vi "Z_plant.vi"(4 "u":dbl format="%#_13g") -> (1 "y":dbl)   [LabVIEW 2015]
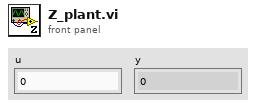
[diagram p1: front panel]
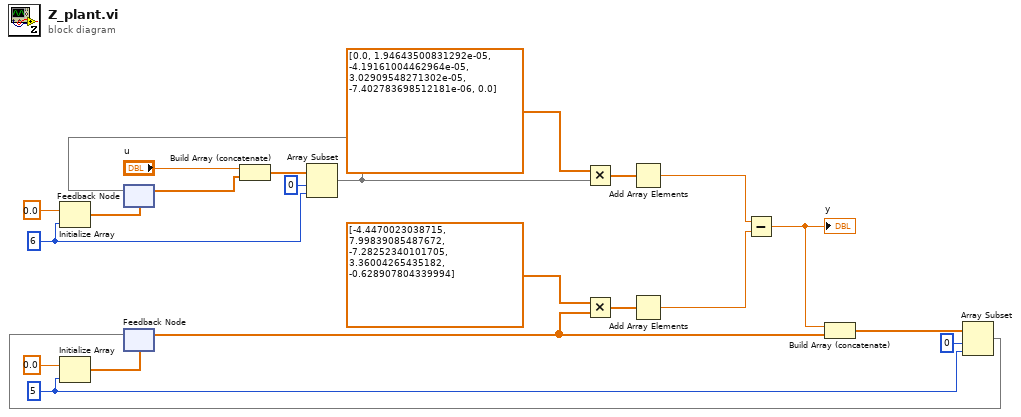
[diagram p0: block diagram]
diagram:
  w8 = 5 ("dimension size")
  w17 = 6 ("dimension size")
  n1 = Initialize Array(0.0 ("element"), w17) -> (w16:dbl[])
  n2 = Initialize Array(0.0 ("element"), w8) -> (w11:dbl[])
  n3 = feedback #1(w16) -> (w21:dbl[])
  n4 = feedback #2(w11) -> (w14:dbl[])
  n5 = Build Array (concatenate)("u", w21) -> (w20:dbl[])
  n6 = Array Subset(array=w20, index=0, length=w17) -> (w15:dbl[])
  n7 = feedback-in #1(w15) -> ()
  n8 = Multiply(x=dbl[] [0.0, 1.94643500831292e-05, -4.19161004462964e-05, 3.02909548271302e-05, -7.402783698512181e-06, 0.0] ("Qd"), y=w15) -> (x*y=w6:dbl[])
  n9 = Multiply(x=dbl[] [-4.4470023038715, 7.99839085487672, -7.28252340101705, 3.36004265435182, -0.628907804339994] ("Qd"), y=w14) -> (x*y=w13:dbl[])
  n10 = Add Array Elements(numeric array=w6) -> (sum=w5:dbl)
  n11 = Add Array Elements(numeric array=w13) -> (sum=w4:dbl)
  n12 = Subtract(x=w5, y=w4) -> (x-y=w3:dbl)
  "y" <- w3
  n13 = Build Array (concatenate)(w3, w14) -> (w10:dbl[])
  n14 = Array Subset(array=w10, index=0, length=w8) -> (w7:dbl[])
  n15 = feedback-in #2(w7) -> ()
